vi "AFT Filtered-X Filter Signal and Update Coefficients.vi"(6 "step size":dbl=-1.0, 7 "reset? (F)":bool, 8 "error in (no error)":errorcluster, 9 "e(n)":dbl, 10 "x(n)":dbl, 11 "filtered-x adaptive filter in":refnum<k20>) -> (0 "error out":errorcluster, 2 "y(n)":dbl, 3 "filtered-x adaptive filter out":refnum<k20>)   [LabVIEW 2017, in "NI_AdaptiveFilter.lvlib"]
doc: "Processes an input signal with an adaptive filter you create by using the AFT Create FIR Filtered-X LMS or AFT Create FIR Normalized Filtered-X LMS VI."
uses:
  <vilib>/addons/Adaptive Filters/NI_AdaptiveFilter.lvlib
  <resource>/AdaptiveFilters.dll
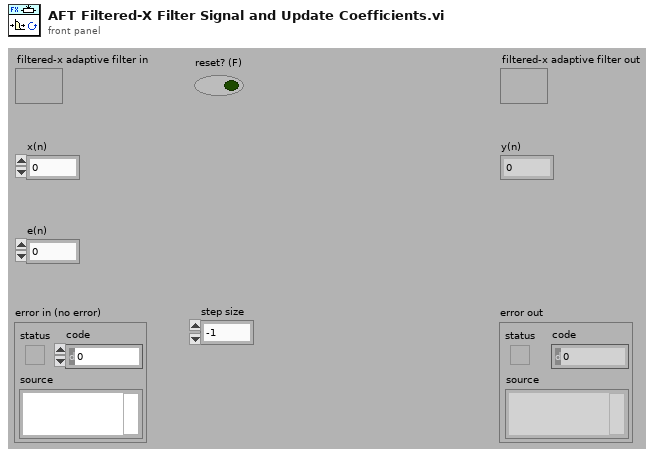
[diagram p1: front panel]
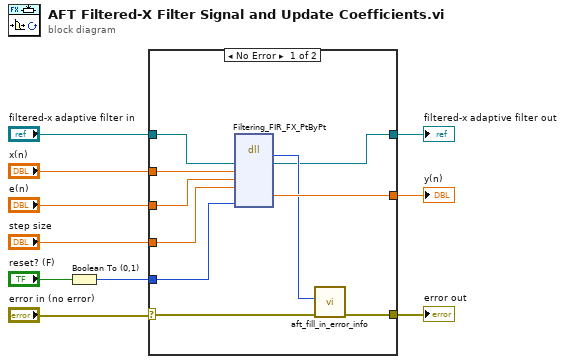
[diagram p0: block diagram]
diagram:
  n1 = Boolean To (0,1)(Boolean="reset? (F)") -> (0, 1=w5:i16)
  n2 = case shown="No Error" "error in (no error)" {
    selector: "error in (no error)" -> [w17 w22]
    tunnel: [w15 w22] -> w10
    tunnel: "filtered-x adaptive filter in" -> [w12 w21]
    tunnel: "x(n)" -> [w20 _]
    tunnel: "e(n)" -> [w19 _]
    tunnel: [w18 _] -> w7
    tunnel: [w11 w21] -> w1
    tunnel: w5 -> [w14 _]
    tunnel: "step size" -> [w13 _]
    frame No Error {
      n3 = dll-call lib="C:/Program Files/National Instruments/LabVIEW 2017/resource/AdaptiveFilters.dll" fn="Filtering_FIR_FX_PtByPt"("pSession"=w12, "x"=w20, "e"=w19, "mu"=w13, "reset"=w14) -> ("err"=w16:i32, "pSession"=w11:refnum<k20>, "y"=w18:dbl)  [unwired: 7 in, 3 out]
      n4 = call <vilib>:"aft_fill_in_error_info.vi"("error in"=w17, "status code"=w16) -> ("error out"=w15:errorcluster)  [unwired: 2 in, 7 out]
    }
    frame Error {
    }
  }
  "error out" <- w10
  "y(n)" <- w7
  "filtered-x adaptive filter out" <- w1
